vi "BMU参数读取-Auto.vi"(7 "Socket":dbl, 8 "CAN端口":u16(ring), 9 "设备索引号":u16(ring), 10 "CAN卡类型":u32(ring)=21, 11 "从板号":u8=1) -> (3 "成功?":bool)   [LabVIEW 2013] (continued)
                n2798 = global read "功能码全局.vi" "主板项目信息5"() -> (w4409:bool[])
                n2799 = global read "功能码全局.vi" "主板项目信息6"() -> (w4407:bool[])
                n2800 = Index Array(array=w4409, index=4 ("索引")) -> (element=w4405:bool)
                n2801 = Index Array(array=w4407, index=5 ("索引")) -> (element=w4406:bool)
                n2802 = Not(x=w4415) -> (.not. x?=w4414:bool)
              }
              frame "温度起始值" {
                w4451 = 2
                w4453 = FALSE
                n2803 = property on="电池实际容量(A)" class="DigNum (严格)"("Disabled"=w4451) -> ()  [unwired: 2 in, 2 out]
                n2804 = property on="使用者" class="DigNum (严格)"("Disabled"=w4451) -> ()  [unwired: 2 in, 2 out]
                n2805 = property on="SOH(%)" class="DigNum (严格)"("Disabled"=w4451) -> ()  [unwired: 2 in, 2 out]
                n2806 = property on="电池额定容量(A)" class="DigNum (严格)"("Disabled"=w4451) -> ()  [unwired: 2 in, 2 out]
                n2807 = property on="SOC(%)" class="DigNum (严格)"("Disabled"=w4451) -> ()  [unwired: 2 in, 2 out]
                n2808 = local read "从板个数"() -> (w4449:dbl)
                n2809 = property on="系统时钟" class="Str"("Disabled"=w4451) -> ()  [unwired: 2 in, 2 out]
                n2810 = property on="配置文件版本" class="Str"("Disabled"=w4451) -> ()  [unwired: 2 in, 2 out]
                n2811 = property on="车架(牌)号" class="Str"("Disabled"=w4451) -> ()  [unwired: 2 in, 2 out]
                n2812 = property on="产品编号" class="Str"("Disabled"=w4451) -> ()  [unwired: 2 in, 2 out]
                n2813 = control-ref of="项目信息"() -> (w4450:refnum<vi>)
                n2814 = stacked-sequence {
                  tunnel: w4450 -> [w4462 w4465 w4478]
                  tunnel: w4449 -> [w4455 w4464 w4477]
                  frame #0 {
                    n2815 = Multiply(x=w4455, y=3.0) -> (x*y=w4457:dbl)
                    n2816 = Compound Arithmetic op=ADD(23.0 ("值"), w4457) -> (w4459:dbl)
                    n2817 = Bundle(w4459, 0) -> (w4461:cluster{dbl, i32})  [unwired: 1 out]
                    n2818 = property class="Tbl (严格)"(reference=w4462, "Index Values"=w4461) -> ()  [unwired: 1 in, 2 out]
                  }
                  frame #1 {
                    n2819 = for {
                      N: 10 -> [_]
                      tunnel: w4465 -> [w4475]
                      tunnel: w4464 -> [w4470]
                      i -> [w4469]
                      n2820 = Multiply(x=4.0, y=w4470) -> (x*y=w4467:dbl)
                      n2821 = Compound Arithmetic op=ADD(24.0 ("值"), w4467, w4469) -> (w4472:dbl)
                      n2822 = Bundle(w4472, 0) -> (w4474:cluster{dbl, i32})  [unwired: 1 out]
                      n2823 = property class="Tbl (严格)"(reference=w4475, "Active Cell"=w4474, "Cell BG Color"=u32 16448250) -> ()  [unwired: 1 in, 2 out]
                    }
                  }
                  frame #2 {
                    n2824 = Increment(x=w4477) -> (x+1=w4476:dbl)
                    n2825 = for {
                      N: w4476 -> [_]
                      tunnel: w4478 -> [w4488]
                      tunnel: w4477 -> [w4483]
                      i -> [w4482]
                      n2826 = Multiply(x=3.0, y=w4483) -> (x*y=w4480:dbl)
                      n2827 = Compound Arithmetic op=ADD(23.0 ("值"), w4480, w4482) -> (w4485:dbl)
                      n2828 = Bundle(w4485, 0) -> (w4487:cluster{dbl, i32})  [unwired: 1 out]
                      n2829 = property class="Tbl (严格)"(reference=w4488, "Active Cell"=w4487, "Cell BG Color"=u32 6618880) -> ()  [unwired: 1 in, 2 out]
                    }
                  }
                }
                n2830 = Select(t=0, s=w4440, f=1) -> (s? t:f=w4439:i32)
                n2831 = property on="从板个数" class="DigNum (严格)"("NumText.BGColor"=u32 13816530) -> ()  [unwired: 2 in, 2 out]
                n2832 = property on="项目信息" class="Tbl (严格)"("Disabled"=w4439) -> ()  [unwired: 2 in, 2 out]
                n2833 = global read "功能码全局.vi" "主板项目信息5"() -> (w4447:bool[])
                n2834 = global read "功能码全局.vi" "主板项目信息6"() -> (w4445:bool[])
                n2835 = Index Array(array=w4447, index=5 ("索引")) -> (element=w4444:bool)
                n2836 = Index Array(array=w4445, index=6 ("索引")) -> (element=w4443:bool)
                n2837 = Not(x=w4453) -> (.not. x?=w4452:bool)
              }
              frame "保险位置" {
                w4501 = 2
                w4503 = FALSE
                n2838 = property on="电池实际容量(A)" class="DigNum (严格)"("Disabled"=w4501) -> ()  [unwired: 2 in, 2 out]
                n2839 = property on="使用者" class="DigNum (严格)"("Disabled"=w4501) -> ()  [unwired: 2 in, 2 out]
                n2840 = property on="SOH(%)" class="DigNum (严格)"("Disabled"=w4501) -> ()  [unwired: 2 in, 2 out]
                n2841 = property on="电池额定容量(A)" class="DigNum (严格)"("Disabled"=w4501) -> ()  [unwired: 2 in, 2 out]
                n2842 = property on="SOC(%)" class="DigNum (严格)"("Disabled"=w4501) -> ()  [unwired: 2 in, 2 out]
                n2843 = local read "从板个数"() -> (w4499:dbl)
                n2844 = property on="系统时钟" class="Str"("Disabled"=w4501) -> ()  [unwired: 2 in, 2 out]
                n2845 = property on="配置文件版本" class="Str"("Disabled"=w4501) -> ()  [unwired: 2 in, 2 out]
                n2846 = property on="车架(牌)号" class="Str"("Disabled"=w4501) -> ()  [unwired: 2 in, 2 out]
                n2847 = property on="产品编号" class="Str"("Disabled"=w4501) -> ()  [unwired: 2 in, 2 out]
                n2848 = control-ref of="项目信息"() -> (w4500:refnum<vi>)
                n2849 = stacked-sequence {
                  tunnel: w4500 -> [w4512 w4515]
                  tunnel: w4499 -> [w4505 w4514]
                  frame #0 {
                    n2850 = Multiply(x=w4505, y=4.0) -> (x*y=w4507:dbl)
                    n2851 = Compound Arithmetic op=ADD(24.0 ("值"), w4507) -> (w4509:dbl)
                    n2852 = Bundle(w4509, 0) -> (w4511:cluster{dbl, i32})  [unwired: 1 out]
                    n2853 = property class="Tbl (严格)"(reference=w4512, "Index Values"=w4511) -> ()  [unwired: 1 in, 2 out]
                  }
                  frame #1 {
                    n2854 = for {
                      N: 20 -> [_]
                      tunnel: w4515 -> [w4525]
                      tunnel: w4514 -> [w4520]
                      i -> [w4519]
                      n2855 = Multiply(x=4.0, y=w4520) -> (x*y=w4517:dbl)
                      n2856 = Compound Arithmetic op=ADD(24.0 ("值"), w4517, w4519) -> (w4522:dbl)
                      n2857 = Bundle(w4522, 0) -> (w4524:cluster{dbl, i32})  [unwired: 1 out]
                      n2858 = property class="Tbl (严格)"(reference=w4525, "Active Cell"=w4524, "Cell BG Color"=u32 6618880) -> ()  [unwired: 1 in, 2 out]
                    }
                  }
                }
                n2859 = property on="从板个数" class="DigNum (严格)"("NumText.BGColor"=u32 13816530) -> ()  [unwired: 2 in, 2 out]
                n2860 = Select(t=0, s=w4492, f=1) -> (s? t:f=w4490:i32)
                n2861 = global read "功能码全局.vi" "主板项目信息4"() -> (w4497:bool[])
                n2862 = property on="项目信息" class="Tbl (严格)"("Disabled"=w4490) -> ()  [unwired: 2 in, 2 out]
                n2863 = Index Array(array=w4497, index #1=5 ("索引"), index #2=6 ("索引")) -> (element #1=w4495:bool, element #2=w4494:bool)
                n2864 = Not(x=w4503) -> (.not. x?=w4502:bool)
              }
              frame "SOC" {
                w4536 = 2
                w4538 = FALSE
                n2865 = property on="电池实际容量(A)" class="DigNum (严格)"("Disabled"=w4536) -> ()  [unwired: 2 in, 2 out]
                n2866 = property on="使用者" class="DigNum (严格)"("Disabled"=w4536) -> ()  [unwired: 2 in, 2 out]
                n2867 = property on="SOH(%)" class="DigNum (严格)"("Disabled"=w4536) -> ()  [unwired: 2 in, 2 out]
                n2868 = property on="电池额定容量(A)" class="DigNum (严格)"("Disabled"=w4536) -> ()  [unwired: 2 in, 2 out]
                n2869 = property on="从板个数" class="DigNum (严格)"("NumText.BGColor"=u32 13816530) -> ()  [unwired: 2 in, 2 out]
                n2870 = property on="系统时钟" class="Str"("Disabled"=w4536) -> ()  [unwired: 2 in, 2 out]
                n2871 = property on="配置文件版本" class="Str"("Disabled"=w4536) -> ()  [unwired: 2 in, 2 out]
                n2872 = property on="车架(牌)号" class="Str"("Disabled"=w4536) -> ()  [unwired: 2 in, 2 out]
                n2873 = property on="项目信息" class="Tbl (严格)"("Disabled"=w4536) -> ()  [unwired: 2 in, 2 out]
                n2874 = property on="产品编号" class="Str"("Disabled"=w4536) -> ()  [unwired: 2 in, 2 out]
                n2875 = Select(t=0, s=w4528, f=0) -> (s? t:f=w4527:i32)
                n2876 = property on="SOC(%)" class="DigNum (严格)"("Disabled"=w4527) -> ()  [unwired: 2 in, 2 out]
                n2877 = property on="项目信息2" class="Clust (严格)"("DisabledEnum"=w4527) -> ()  [unwired: 2 in, 2 out]
                n2878 = global read "功能码全局.vi" "主板项目信息7"() -> (w4534:bool[])
                n2879 = Index Array(array=w4534, index #1=2 ("索引"), index #2=5 ("索引")) -> (element #1=w4532:bool, element #2=w4531:bool)
                n2880 = Not(x=w4538) -> (.not. x?=w4537:bool)
              }
              frame "电池额定实际容量" {
                w4550 = 2
                w4552 = FALSE
                n2881 = property on="使用者" class="DigNum (严格)"("Disabled"=w4550) -> ()  [unwired: 2 in, 2 out]
                n2882 = property on="SOH(%)" class="DigNum (严格)"("Disabled"=w4550) -> ()  [unwired: 2 in, 2 out]
                n2883 = property on="SOC(%)" class="DigNum (严格)"("Disabled"=w4550) -> ()  [unwired: 2 in, 2 out]
                n2884 = property on="从板个数" class="DigNum (严格)"("NumText.BGColor"=u32 13816530) -> ()  [unwired: 2 in, 2 out]
                n2885 = property on="系统时钟" class="Str"("Disabled"=w4550) -> ()  [unwired: 2 in, 2 out]
                n2886 = property on="配置文件版本" class="Str"("Disabled"=w4550) -> ()  [unwired: 2 in, 2 out]
                n2887 = property on="车架(牌)号" class="Str"("Disabled"=w4550) -> ()  [unwired: 2 in, 2 out]
                n2888 = property on="项目信息" class="Tbl (严格)"("Disabled"=w4550) -> ()  [unwired: 2 in, 2 out]
                n2889 = property on="产品编号" class="Str"("Disabled"=w4550) -> ()  [unwired: 2 in, 2 out]
                n2890 = Select(t=0, s=w4542, f=1) -> (s? t:f=w4541:i32)
                n2891 = property on="电池实际容量(A)" class="DigNum (严格)"("Disabled"=w4541) -> ()  [unwired: 2 in, 2 out]
                n2892 = property on="电池额定容量(A)" class="DigNum (严格)"("Disabled"=w4541) -> ()  [unwired: 2 in, 2 out]
                n2893 = property on="项目信息2" class="Clust (严格)"("DisabledEnum"=w4541) -> ()  [unwired: 2 in, 2 out]
                n2894 = global read "功能码全局.vi" "主板项目信息7"() -> (w4548:bool[])
                n2895 = Index Array(array=w4548, index #1=3 ("索引"), index #2=6 ("索引")) -> (element #1=w4546:bool, element #2=w4545:bool)
                n2896 = Not(x=w4552) -> (.not. x?=w4551:bool)
              }
              frame "配置文件版本" {
                w4565 = 2
                w4567 = FALSE
                n2897 = property on="使用者" class="DigNum (严格)"("Disabled"=w4565) -> ()  [unwired: 2 in, 2 out]
                n2898 = property on="SOH(%)" class="DigNum (严格)"("Disabled"=w4565) -> ()  [unwired: 2 in, 2 out]
                n2899 = property on="SOC(%)" class="DigNum (严格)"("Disabled"=w4565) -> ()  [unwired: 2 in, 2 out]
                n2900 = property on="电池实际容量(A)" class="DigNum (严格)"("Disabled"=w4565) -> ()  [unwired: 2 in, 2 out]
                n2901 = property on="从板个数" class="DigNum (严格)"("NumText.BGColor"=u32 13816530) -> ()  [unwired: 2 in, 2 out]
                n2902 = property on="电池额定容量(A)" class="DigNum (严格)"("Disabled"=w4565) -> ()  [unwired: 2 in, 2 out]
                n2903 = property on="系统时钟" class="Str"("Disabled"=w4565) -> ()  [unwired: 2 in, 2 out]
                n2904 = property on="车架(牌)号" class="Str"("Disabled"=w4565) -> ()  [unwired: 2 in, 2 out]
                n2905 = property on="项目信息" class="Tbl (严格)"("Disabled"=w4565) -> ()  [unwired: 2 in, 2 out]
                n2906 = property on="产品编号" class="Str"("Disabled"=w4565) -> ()  [unwired: 2 in, 2 out]
                n2907 = Select(t=0, s=w4556, f=1) -> (s? t:f=w4555:i32)
                n2908 = property on="项目信息2" class="Clust (严格)"("DisabledEnum"=w4555) -> ()  [unwired: 2 in, 2 out]
                n2909 = property on="配置文件版本" class="Str"("Disabled"=w4555) -> ()  [unwired: 2 in, 2 out]
                n2910 = global read "功能码全局.vi" "主板项目信息5"() -> (w4563:bool[])
                n2911 = global read "功能码全局.vi" "主板项目信息6"() -> (w4562:bool[])
                n2912 = Index Array(array=w4563, index=6 ("索引")) -> (element=w4560:bool)
                n2913 = Index Array(array=w4562, index=7 ("索引")) -> (element=w4559:bool)
                n2914 = Not(x=w4567) -> (.not. x?=w4566:bool)
              }
              frame "参数修改记录" {
                w4580 = 2
                w4582 = FALSE
                n2915 = property on="SOH(%)" class="DigNum (严格)"("Disabled"=w4580) -> ()  [unwired: 2 in, 2 out]
                n2916 = property on="SOC(%)" class="DigNum (严格)"("Disabled"=w4580) -> ()  [unwired: 2 in, 2 out]
                n2917 = property on="电池实际容量(A)" class="DigNum (严格)"("Disabled"=w4580) -> ()  [unwired: 2 in, 2 out]
                n2918 = property on="电池额定容量(A)" class="DigNum (严格)"("Disabled"=w4580) -> ()  [unwired: 2 in, 2 out]
                n2919 = property on="从板个数" class="DigNum (严格)"("NumText.BGColor"=u32 13816530) -> ()  [unwired: 2 in, 2 out]
                n2920 = property on="系统时钟" class="Str"("Disabled"=w4580) -> ()  [unwired: 2 in, 2 out]
                n2921 = property on="车架(牌)号" class="Str"("Disabled"=w4580) -> ()  [unwired: 2 in, 2 out]
                n2922 = property on="配置文件版本" class="Str"("Disabled"=w4580) -> ()  [unwired: 2 in, 2 out]
                n2923 = property on="项目信息" class="Tbl (严格)"("Disabled"=w4580) -> ()  [unwired: 2 in, 2 out]
                n2924 = property on="产品编号" class="Str"("Disabled"=w4580) -> ()  [unwired: 2 in, 2 out]
                n2925 = Select(t=0, s=w4571, f=1) -> (s? t:f=w4570:i32)
                n2926 = property on="使用者" class="DigNum (严格)"("Disabled"=w4570) -> ()  [unwired: 2 in, 2 out]
                n2927 = property on="项目信息2" class="Clust (严格)"("DisabledEnum"=w4570) -> ()  [unwired: 2 in, 2 out]
                n2928 = global read "功能码全局.vi" "主板项目信息7"() -> (w4577:bool[])
                n2929 = global read "功能码全局.vi" "主板项目信息5"() -> (w4578:bool[])
                n2930 = Index Array(array=w4577, index=0 ("索引")) -> (element=w4575:bool)
                n2931 = Index Array(array=w4578, index=7 ("索引")) -> (element=w4574:bool)
                n2932 = Not(x=w4582) -> (.not. x?=w4581:bool)
              }
              frame "车牌号" {
                w4595 = 2
                w4597 = FALSE
                n2933 = property on="SOH(%)" class="DigNum (严格)"("Disabled"=w4595) -> ()  [unwired: 2 in, 2 out]
                n2934 = property on="使用者" class="DigNum (严格)"("Disabled"=w4595) -> ()  [unwired: 2 in, 2 out]
                n2935 = property on="SOC(%)" class="DigNum (严格)"("Disabled"=w4595) -> ()  [unwired: 2 in, 2 out]
                n2936 = property on="电池实际容量(A)" class="DigNum (严格)"("Disabled"=w4595) -> ()  [unwired: 2 in, 2 out]
                n2937 = property on="电池额定容量(A)" class="DigNum (严格)"("Disabled"=w4595) -> ()  [unwired: 2 in, 2 out]
                n2938 = property on="从板个数" class="DigNum (严格)"("NumText.BGColor"=u32 13816530) -> ()  [unwired: 2 in, 2 out]
                n2939 = property on="系统时钟" class="Str"("Disabled"=w4595) -> ()  [unwired: 2 in, 2 out]
                n2940 = property on="配置文件版本" class="Str"("Disabled"=w4595) -> ()  [unwired: 2 in, 2 out]
                n2941 = property on="项目信息" class="Tbl (严格)"("Disabled"=w4595) -> ()  [unwired: 2 in, 2 out]
                n2942 = property on="产品编号" class="Str"("Disabled"=w4595) -> ()  [unwired: 2 in, 2 out]
                n2943 = Select(t=0, s=w4586, f=1) -> (s? t:f=w4585:i32)
                n2944 = property on="车架(牌)号" class="Str"("Disabled"=w4585) -> ()  [unwired: 2 in, 2 out]
                n2945 = property on="项目信息2" class="Clust (严格)"("DisabledEnum"=w4585) -> ()  [unwired: 2 in, 2 out]
                n2946 = global read "功能码全局.vi" "主板项目信息7"() -> (w4592:bool[])
                n2947 = global read "功能码全局.vi" "主板项目信息6"() -> (w4593:bool[])
                n2948 = Index Array(array=w4592, index=1 ("索引")) -> (element=w4590:bool)
                n2949 = Index Array(array=w4593, index=0 ("索引")) -> (element=w4589:bool)
                n2950 = Not(x=w4597) -> (.not. x?=w4596:bool)
              }
              frame "SOH" {
                w4609 = 2
                w4611 = FALSE
                n2951 = property on="使用者" class="DigNum (严格)"("Disabled"=w4609) -> ()  [unwired: 2 in, 2 out]
                n2952 = property on="SOC(%)" class="DigNum (严格)"("Disabled"=w4609) -> ()  [unwired: 2 in, 2 out]
                n2953 = property on="电池实际容量(A)" class="DigNum (严格)"("Disabled"=w4609) -> ()  [unwired: 2 in, 2 out]
                n2954 = property on="电池额定容量(A)" class="DigNum (严格)"("Disabled"=w4609) -> ()  [unwired: 2 in, 2 out]
                n2955 = property on="从板个数" class="DigNum (严格)"("NumText.BGColor"=u32 13816530) -> ()  [unwired: 2 in, 2 out]
                n2956 = property on="系统时钟" class="Str"("Disabled"=w4609) -> ()  [unwired: 2 in, 2 out]
                n2957 = property on="配置文件版本" class="Str"("Disabled"=w4609) -> ()  [unwired: 2 in, 2 out]
                n2958 = property on="项目信息" class="Tbl (严格)"("Disabled"=w4609) -> ()  [unwired: 2 in, 2 out]
                n2959 = property on="产品编号" class="Str"("Disabled"=w4609) -> ()  [unwired: 2 in, 2 out]
                n2960 = property on="车架(牌)号" class="Str"("Disabled"=w4609) -> ()  [unwired: 2 in, 2 out]
                n2961 = Select(t=0, s=w4601, f=1) -> (s? t:f=w4600:i32)
                n2962 = property on="项目信息2" class="Clust (严格)"("DisabledEnum"=w4600) -> ()  [unwired: 2 in, 2 out]
                n2963 = property on="SOH(%)" class="DigNum (严格)"("Disabled"=w4600) -> ()  [unwired: 2 in, 2 out]
                n2964 = global read "功能码全局.vi" "主板项目信息7"() -> (w4608:bool[])
                n2965 = Index Array(array=w4608, index #1=4 ("索引"), index #2=7 ("索引")) -> (element #1=w4605:bool, element #2=w4604:bool)
                n2966 = Not(x=w4611) -> (.not. x?=w4610:bool)
              }
              frame "SOC过低(2)", "SOC过高(2)", "SOH过低(2)", "充电电流过高(2)", "单体电压过低(2)", "单体电压过高(2)", "单组电压不均衡(2)", "单组温度不均衡(2)", "二级故障阀值", "放电电流过高(2)", "极柱温度过高(2)", "内阻过大(2)", "温度过低(2)", "温度过高(2)", "整组电压不均衡(2)", "整组温度不均衡(2)", "总电压过低(2)", "总电压过高(2)" {
                w4623 = FALSE
                n2967 = property on="从板个数" class="DigNum (严格)"("NumText.BGColor"=u32 13816530) -> ()  [unwired: 2 in, 2 out]
                n2968 = Select(t=0, s=w4615, f=1) -> (s? t:f=w4614:i32)
                n2969 = property on="一级故障 2" class="Clust (严格)"("DisabledEnum"=w4614) -> ()  [unwired: 2 in, 2 out]
                n2970 = global read "功能码全局.vi" "主板故障阀值9"() -> (w4621:bool[])
                n2971 = Index Array(array=w4621, index #1=3 ("索引"), index #2=6 ("索引")) -> (element #1=w4619:bool, element #2=w4618:bool)
                n2972 = Not(x=w4623) -> (.not. x?=w4624:bool)
              }
              frame "SOC过低(3)", "SOC过高(3)", "SOH过低(3)", "充电电流过高(3)", "单体电压过低(3)", "单体电压过高(3)", "单组电压不均衡(3)", "单组温度不均衡(3)", "放电电流过高(3)", "极柱温度过高(3)", "内阻过大(3)", "三级故障阀值", "温度过低(3)", "温度过高(3)", "整组电压不均衡(3)", "整组温度不均衡(3)", "总电压过低(3)", "总电压过高(3)" {
                w4637 = FALSE
                n2973 = property on="从板个数" class="DigNum (严格)"("NumText.BGColor"=u32 13816530) -> ()  [unwired: 2 in, 2 out]
                n2974 = Select(t=0, s=w4628, f=1) -> (s? t:f=w4627:i32)
                n2975 = property on="一级故障 3" class="Clust (严格)"("DisabledEnum"=w4627) -> ()  [unwired: 2 in, 2 out]
                n2976 = global read "功能码全局.vi" "主板故障阀值9"() -> (w4634:bool[])
                n2977 = Index Array(array=w4634, index #1=4 ("索引"), index #2=7 ("索引")) -> (element #1=w4632:bool, element #2=w4631:bool)
                n2978 = Not(x=w4637) -> (.not. x?=w4636:bool)
              }
              frame "SOC过低", "SOC过高", "SOH过低", "充电电流过高", "单体电压过低", "单体电压过高", "单组电压不均衡", "单组温度不均衡", "放电电流过高", "极柱温度过高", "内阻过大", "温度过低", "温度过高", "一级故障阀值", "整组电压不均衡", "整组温度不均衡", "总电压过低", "总电压过高" {
                w4650 = FALSE
                n2979 = Select(t=0, s=w4641, f=1) -> (s? t:f=w4640:i32)
                n2980 = property on="从板个数" class="DigNum (严格)"("NumText.BGColor"=u32 13816530) -> ()  [unwired: 2 in, 2 out]
                n2981 = property on="一级故障" class="Clust (严格)"("DisabledEnum"=w4640) -> ()  [unwired: 2 in, 2 out]
                n2982 = global read "功能码全局.vi" "主板故障阀值9"() -> (w4647:bool[])
                n2983 = Index Array(array=w4647, index #1=2 ("索引"), index #2=5 ("索引")) -> (element #1=w4645:bool, element #2=w4644:bool)
                n2984 = Not(x=w4650) -> (.not. x?=w4649:bool)
              }
              frame "充电控制参数", "电流步长", "最大允许充电电流", "最大允许充电温度", "最大允许单体电压", "最大允许总电压", "最小允许充电电流", "最小允许充电温度", "最小允许单体电压" {
                w4653 = 2
                w4664 = FALSE
                n2985 = property on="从板个数" class="DigNum (严格)"("NumText.BGColor"=u32 13816530) -> ()  [unwired: 2 in, 2 out]
                n2986 = property on="风机开启温度" class="DigNum (严格)"("Disabled"=w4653) -> ()  [unwired: 2 in, 2 out]
                n2987 = property on="风机关闭温度" class="DigNum (严格)"("Disabled"=w4653) -> ()  [unwired: 2 in, 2 out]
                n2988 = property on="加热开启温度" class="DigNum (严格)"("Disabled"=w4653) -> ()  [unwired: 2 in, 2 out]
                n2989 = property on="加热关闭温度" class="DigNum (严格)"("Disabled"=w4653) -> ()  [unwired: 2 in, 2 out]
                n2990 = property on="风机开启温差" class="DigNum (严格)"("Disabled"=w4653) -> ()  [unwired: 2 in, 2 out]
                n2991 = property on="风机关闭温差" class="DigNum (严格)"("Disabled"=w4653) -> ()  [unwired: 2 in, 2 out]
                n2992 = property on="加热控制参数" class="Clust (严格)"("DisabledEnum"=w4653) -> ()  [unwired: 2 in, 2 out]
                n2993 = Select(t=0, s=w4655, f=1) -> (s? t:f=w4654:i32)
                n2994 = property on="最大允许总电压" class="DigNum (严格)"("Disabled"=w4654) -> ()  [unwired: 2 in, 2 out]
                n2995 = property on="最大允许充电温度" class="DigNum (严格)"("Disabled"=w4654) -> ()  [unwired: 2 in, 2 out]
                n2996 = property on="最小允许充电温度" class="DigNum (严格)"("Disabled"=w4654) -> ()  [unwired: 2 in, 2 out]
                n2997 = property on="电流步长" class="DigNum (严格)"("Disabled"=w4654) -> ()  [unwired: 2 in, 2 out]
                n2998 = property on="最大允许单体电压" class="DigNum (严格)"("Disabled"=w4654) -> ()  [unwired: 2 in, 2 out]
                n2999 = property on="最小允许单体电压" class="DigNum (严格)"("Disabled"=w4654) -> ()  [unwired: 2 in, 2 out]
                n3000 = property on="最大允许充电电流" class="DigNum (严格)"("Disabled"=w4654) -> ()  [unwired: 2 in, 2 out]
                n3001 = property on="最小允许充电电流" class="DigNum (严格)"("Disabled"=w4654) -> ()  [unwired: 2 in, 2 out]
                n3002 = global read "功能码全局.vi" "主板控制类信息10"() -> (w4661:bool[])
                n3003 = Index Array(array=w4661, index #1=5 ("索引"), index #2=7 ("索引")) -> (element #1=w4659:bool, element #2=w4658:bool)
                n3004 = Not(x=w4664) -> (.not. x?=w4663:bool)
              }
              frame "风机关闭温差", "风机关闭温度", "风机开启温差", "风机开启温度", "加热关闭温差", "加热关闭温度", "加热开启温度", "加热控制参数" {
                w4676 = 2
                w4678 = FALSE
                n3005 = Select(t=0, s=w4668, f=1) -> (s? t:f=w4667:i32)
                n3006 = property on="从板个数" class="DigNum (严格)"("NumText.BGColor"=u32 13816530) -> ()  [unwired: 2 in, 2 out]
                n3007 = property on="加热控制参数" class="Clust (严格)"("DisabledEnum"=w4667) -> ()  [unwired: 2 in, 2 out]
                n3008 = property on="风机开启温度" class="DigNum (严格)"("Disabled"=w4667) -> ()  [unwired: 2 in, 2 out]
                n3009 = property on="风机关闭温度" class="DigNum (严格)"("Disabled"=w4667) -> ()  [unwired: 2 in, 2 out]
                n3010 = property on="加热开启温度" class="DigNum (严格)"("Disabled"=w4667) -> ()  [unwired: 2 in, 2 out]
                n3011 = property on="加热关闭温度" class="DigNum (严格)"("Disabled"=w4667) -> ()  [unwired: 2 in, 2 out]
                n3012 = property on="风机开启温差" class="DigNum (严格)"("Disabled"=w4667) -> ()  [unwired: 2 in, 2 out]
                n3013 = property on="风机关闭温差" class="DigNum (严格)"("Disabled"=w4667) -> ()  [unwired: 2 in, 2 out]
                n3014 = property on="最大允许总电压" class="DigNum (严格)"("Disabled"=w4676) -> ()  [unwired: 2 in, 2 out]
                n3015 = property on="最大允许充电温度" class="DigNum (严格)"("Disabled"=w4676) -> ()  [unwired: 2 in, 2 out]
                n3016 = property on="最小允许充电温度" class="DigNum (严格)"("Disabled"=w4676) -> ()  [unwired: 2 in, 2 out]
                n3017 = property on="电流步长" class="DigNum (严格)"("Disabled"=w4676) -> ()  [unwired: 2 in, 2 out]
                n3018 = property on="最大允许单体电压" class="DigNum (严格)"("Disabled"=w4676) -> ()  [unwired: 2 in, 2 out]
                n3019 = property on="最小允许单体电压" class="DigNum (严格)"("Disabled"=w4676) -> ()  [unwired: 2 in, 2 out]
                n3020 = property on="最大允许充电电流" class="DigNum (严格)"("Disabled"=w4676) -> ()  [unwired: 2 in, 2 out]
                n3021 = property on="最小允许充电电流" class="DigNum (严格)"("Disabled"=w4676) -> ()  [unwired: 2 in, 2 out]
                n3022 = global read "功能码全局.vi" "主板控制类信息10"() -> (w4674:bool[])
                n3023 = Index Array(array=w4674, index #1=4 ("索引"), index #2=6 ("索引")) -> (element #1=w4672:bool, element #2=w4671:bool)
                n3024 = Not(x=w4678) -> (.not. x?=w4677:bool)
              }
              frame "电池信息" {
                w4691 = FALSE
                n3025 = Select(t=0, s=w4682, f=1) -> (s? t:f=w4681:i32)
                n3026 = property on="电池串联" class="DigNum (严格)"("Disabled"=w4681) -> ()  [unwired: 2 in, 2 out]
                n3027 = property on="电池并联" class="DigNum (严格)"("Disabled"=w4681) -> ()  [unwired: 2 in, 2 out]
                n3028 = property on="电池包额定容量" class="DigNum (严格)"("Disabled"=w4681) -> ()  [unwired: 2 in, 2 out]
                n3029 = property on="电池包额定能量(kWh)" class="DigNum (严格)"("Disabled"=w4681) -> ()  [unwired: 2 in, 2 out]
                n3030 = property on="电池包额定总电压" class="DigNum (严格)"("Disabled"=w4681) -> ()  [unwired: 2 in, 2 out]
                n3031 = property on="实际容量" class="DigNum (严格)"("Disabled"=w4681) -> ()  [unwired: 2 in, 2 out]
                n3032 = property on="电池包组号" class="Str"("Disabled"=w4681) -> ()  [unwired: 2 in, 2 out]
                n3033 = property on="电池生产日期" class="Str"("Disabled"=w4681) -> ()  [unwired: 2 in, 2 out]
                n3034 = property on="电池厂家" class="Str"("Disabled"=w4681) -> ()  [unwired: 2 in, 2 out]
                n3035 = property on="电池类型" class="Str"("Disabled"=w4681) -> ()  [unwired: 2 in, 2 out]
                n3036 = property on="累计充电总安时" class="DigNum (严格)"("Disabled"=w4681) -> ()  [unwired: 2 in, 2 out]
                n3037 = property on="累计放电总安时" class="DigNum (严格)"("Disabled"=w4681) -> ()  [unwired: 2 in, 2 out]
                n3038 = property on="电池放空次数" class="DigNum (严格)"("Disabled"=w4681) -> ()  [unwired: 2 in, 2 out]
                n3039 = property on="电池充满次数" class="DigNum (严格)"("Disabled"=w4681) -> ()  [unwired: 2 in, 2 out]
                n3040 = property on="电池充电次数" class="DigNum (严格)"("Disabled"=w4681) -> ()  [unwired: 2 in, 2 out]
                n3041 = property on="电池信息" class="Clust (严格)"("DisabledEnum"=w4681) -> ()  [unwired: 2 in, 2 out]
                n3042 = global read "功能码全局.vi" "主板版本号11"() -> (w4688:bool[])
                n3043 = property on="从板个数" class="DigNum (严格)"("NumText.BGColor"=u32 13816530) -> ()  [unwired: 2 in, 2 out]
                n3044 = Index Array(array=w4688, index #1=0 ("索引"), index #2=1 ("索引")) -> (element #1=w4686:bool, element #2=w4685:bool)
                n3045 = Not(x=w4691) -> (.not. x?=w4690:bool)
              }
              frame "电池信息1" {
                w4703 = 2
                w4705 = FALSE
                n3046 = Select(t=0, s=w4695, f=1) -> (s? t:f=w4694:i32)
                n3047 = property on="电池信息" class="Clust (严格)"("DisabledEnum"=w4694) -> ()  [unwired: 2 in, 2 out]
                n3048 = property on="电池生产日期" class="Str"("Disabled"=w4694) -> ()  [unwired: 2 in, 2 out]
                n3049 = property on="电池厂家" class="Str"("Disabled"=w4694) -> ()  [unwired: 2 in, 2 out]
                n3050 = property on="电池类型" class="Str"("Disabled"=w4694) -> ()  [unwired: 2 in, 2 out]
                n3051 = property on="电池串联" class="DigNum (严格)"("Disabled"=w4694) -> ()  [unwired: 2 in, 2 out]
                n3052 = property on="电池并联" class="DigNum (严格)"("Disabled"=w4694) -> ()  [unwired: 2 in, 2 out]
                n3053 = property on="电池包额定容量" class="DigNum (严格)"("Disabled"=w4694) -> ()  [unwired: 2 in, 2 out]
                n3054 = property on="电池包额定能量(kWh)" class="DigNum (严格)"("Disabled"=w4694) -> ()  [unwired: 2 in, 2 out]
                n3055 = property on="电池包额定总电压" class="DigNum (严格)"("Disabled"=w4694) -> ()  [unwired: 2 in, 2 out]
                n3056 = property on="实际容量" class="DigNum (严格)"("Disabled"=w4694) -> ()  [unwired: 2 in, 2 out]
                n3057 = property on="累计充电总安时" class="DigNum (严格)"("Disabled"=w4703) -> ()  [unwired: 2 in, 2 out]
                n3058 = property on="累计放电总安时" class="DigNum (严格)"("Disabled"=w4703) -> ()  [unwired: 2 in, 2 out]
                n3059 = property on="电池放空次数" class="DigNum (严格)"("Disabled"=w4703) -> ()  [unwired: 2 in, 2 out]
                n3060 = property on="电池充满次数" class="DigNum (严格)"("Disabled"=w4703) -> ()  [unwired: 2 in, 2 out]
                n3061 = property on="电池充电次数" class="DigNum (严格)"("Disabled"=w4703) -> ()  [unwired: 2 in, 2 out]
                n3062 = property on="从板个数" class="DigNum (严格)"("NumText.BGColor"=u32 13816530) -> ()  [unwired: 2 in, 2 out]
                n3063 = property on="电池包组号" class="Str"("Disabled"=w4703) -> ()  [unwired: 2 in, 2 out]
                n3064 = global read "功能码全局.vi" "主板版本号11"() -> (w4701:bool[])
                n3065 = Index Array(array=w4701, index #1=0 ("索引"), index #2=1 ("索引")) -> (element #1=w4699:bool, element #2=w4698:bool)
                n3066 = Not(x=w4705) -> (.not. x?=w4704:bool)
              }
              frame "电池包组号" {
                w4717 = 2
                w4719 = FALSE
                n3067 = property on="电池生产日期" class="Str"("Disabled"=w4717) -> ()  [unwired: 2 in, 2 out]
                n3068 = property on="电池厂家" class="Str"("Disabled"=w4717) -> ()  [unwired: 2 in, 2 out]
                n3069 = property on="电池类型" class="Str"("Disabled"=w4717) -> ()  [unwired: 2 in, 2 out]
                n3070 = property on="电池串联" class="DigNum (严格)"("Disabled"=w4717) -> ()  [unwired: 2 in, 2 out]
                n3071 = property on="电池并联" class="DigNum (严格)"("Disabled"=w4717) -> ()  [unwired: 2 in, 2 out]
                n3072 = property on="电池包额定容量" class="DigNum (严格)"("Disabled"=w4717) -> ()  [unwired: 2 in, 2 out]
                n3073 = property on="电池包额定能量(kWh)" class="DigNum (严格)"("Disabled"=w4717) -> ()  [unwired: 2 in, 2 out]
                n3074 = property on="电池包额定总电压" class="DigNum (严格)"("Disabled"=w4717) -> ()  [unwired: 2 in, 2 out]
                n3075 = property on="实际容量" class="DigNum (严格)"("Disabled"=w4717) -> ()  [unwired: 2 in, 2 out]
                n3076 = property on="从板个数" class="DigNum (严格)"("NumText.BGColor"=u32 13816530) -> ()  [unwired: 2 in, 2 out]
                n3077 = property on="累计充电总安时" class="DigNum (严格)"("Disabled"=w4717) -> ()  [unwired: 2 in, 2 out]
                n3078 = property on="累计放电总安时" class="DigNum (严格)"("Disabled"=w4717) -> ()  [unwired: 2 in, 2 out]
                n3079 = property on="电池放空次数" class="DigNum (严格)"("Disabled"=w4717) -> ()  [unwired: 2 in, 2 out]
                n3080 = property on="电池充满次数" class="DigNum (严格)"("Disabled"=w4717) -> ()  [unwired: 2 in, 2 out]
                n3081 = property on="电池充电次数" class="DigNum (严格)"("Disabled"=w4717) -> ()  [unwired: 2 in, 2 out]
                n3082 = Select(t=0, s=w4709, f=1) -> (s? t:f=w4708:i32)
                n3083 = property on="电池包组号" class="Str"("Disabled"=w4708) -> ()  [unwired: 2 in, 2 out]
                n3084 = property on="电池信息" class="Clust (严格)"("DisabledEnum"=w4708) -> ()  [unwired: 2 in, 2 out]
                n3085 = global read "功能码全局.vi" "主板版本号11"() -> (w4715:bool[])
                n3086 = Index Array(array=w4715, index #1=0 ("索引"), index #2=1 ("索引")) -> (element #1=w4713:bool, element #2=w4712:bool)
                n3087 = Not(x=w4719) -> (.not. x?=w4718:bool)
              }
              frame "充放电安时" {
                w4731 = 2
                w4733 = FALSE
                n3088 = property on="电池生产日期" class="Str"("Disabled"=w4731) -> ()  [unwired: 2 in, 2 out]
                n3089 = property on="电池厂家" class="Str"("Disabled"=w4731) -> ()  [unwired: 2 in, 2 out]
                n3090 = property on="电池类型" class="Str"("Disabled"=w4731) -> ()  [unwired: 2 in, 2 out]
                n3091 = property on="电池串联" class="DigNum (严格)"("Disabled"=w4731) -> ()  [unwired: 2 in, 2 out]
                n3092 = property on="电池并联" class="DigNum (严格)"("Disabled"=w4731) -> ()  [unwired: 2 in, 2 out]
                n3093 = property on="电池包额定容量" class="DigNum (严格)"("Disabled"=w4731) -> ()  [unwired: 2 in, 2 out]
                n3094 = property on="电池包额定能量(kWh)" class="DigNum (严格)"("Disabled"=w4731) -> ()  [unwired: 2 in, 2 out]
                n3095 = property on="电池包额定总电压" class="DigNum (严格)"("Disabled"=w4731) -> ()  [unwired: 2 in, 2 out]
                n3096 = property on="实际容量" class="DigNum (严格)"("Disabled"=w4731) -> ()  [unwired: 2 in, 2 out]
                n3097 = property on="从板个数" class="DigNum (严格)"("NumText.BGColor"=u32 13816530) -> ()  [unwired: 2 in, 2 out]
                n3098 = Select(t=0, s=w4723, f=1) -> (s? t:f=w4722:i32)
                n3099 = property on="电池放空次数" class="DigNum (严格)"("Disabled"=w4731) -> ()  [unwired: 2 in, 2 out]
                n3100 = property on="电池充满次数" class="DigNum (严格)"("Disabled"=w4731) -> ()  [unwired: 2 in, 2 out]
                n3101 = property on="电池充电次数" class="DigNum (严格)"("Disabled"=w4731) -> ()  [unwired: 2 in, 2 out]
                n3102 = property on="电池包组号" class="Str"("Disabled"=w4731) -> ()  [unwired: 2 in, 2 out]
                n3103 = property on="累计充电总安时" class="DigNum (严格)"("Disabled"=w4722) -> ()  [unwired: 2 in, 2 out]
                n3104 = property on="累计放电总安时" class="DigNum (严格)"("Disabled"=w4722) -> ()  [unwired: 2 in, 2 out]
                n3105 = property on="电池信息" class="Clust (严格)"("DisabledEnum"=w4722) -> ()  [unwired: 2 in, 2 out]
                n3106 = global read "功能码全局.vi" "主板版本号11"() -> (w4729:bool[])
                n3107 = Index Array(array=w4729, index #1=0 ("索引"), index #2=1 ("索引")) -> (element #1=w4727:bool, element #2=w4726:bool)
                n3108 = Not(x=w4733) -> (.not. x?=w4732:bool)
              }
              frame "电池充放电次数" {
                w4745 = 2
                w4747 = FALSE
                n3109 = property on="从板个数" class="DigNum (严格)"("NumText.BGColor"=u32 13816530) -> ()  [unwired: 2 in, 2 out]
                n3110 = property on="电池生产日期" class="Str"("Disabled"=w4745) -> ()  [unwired: 2 in, 2 out]
                n3111 = property on="电池厂家" class="Str"("Disabled"=w4745) -> ()  [unwired: 2 in, 2 out]
                n3112 = property on="电池类型" class="Str"("Disabled"=w4745) -> ()  [unwired: 2 in, 2 out]
                n3113 = property on="电池串联" class="DigNum (严格)"("Disabled"=w4745) -> ()  [unwired: 2 in, 2 out]
                n3114 = property on="电池并联" class="DigNum (严格)"("Disabled"=w4745) -> ()  [unwired: 2 in, 2 out]
                n3115 = property on="电池包额定容量" class="DigNum (严格)"("Disabled"=w4745) -> ()  [unwired: 2 in, 2 out]
                n3116 = property on="电池包额定能量(kWh)" class="DigNum (严格)"("Disabled"=w4745) -> ()  [unwired: 2 in, 2 out]
                n3117 = property on="电池包额定总电压" class="DigNum (严格)"("Disabled"=w4745) -> ()  [unwired: 2 in, 2 out]
                n3118 = property on="实际容量" class="DigNum (严格)"("Disabled"=w4745) -> ()  [unwired: 2 in, 2 out]
                n3119 = Select(t=0, s=w4737, f=1) -> (s? t:f=w4736:i32)
                n3120 = property on="电池放空次数" class="DigNum (严格)"("Disabled"=w4736) -> ()  [unwired: 2 in, 2 out]
                n3121 = property on="电池充满次数" class="DigNum (严格)"("Disabled"=w4736) -> ()  [unwired: 2 in, 2 out]
                n3122 = property on="电池充电次数" class="DigNum (严格)"("Disabled"=w4736) -> ()  [unwired: 2 in, 2 out]
                n3123 = property on="累计充电总安时" class="DigNum (严格)"("Disabled"=w4745) -> ()  [unwired: 2 in, 2 out]
                n3124 = property on="累计放电总安时" class="DigNum (严格)"("Disabled"=w4745) -> ()  [unwired: 2 in, 2 out]
                n3125 = property on="电池信息" class="Clust (严格)"("DisabledEnum"=w4736) -> ()  [unwired: 2 in, 2 out]
                n3126 = property on="电池包组号" class="Str"("Disabled"=w4745) -> ()  [unwired: 2 in, 2 out]
                n3127 = global read "功能码全局.vi" "主板版本号11"() -> (w4743:bool[])
                n3128 = Index Array(array=w4743, index #1=0 ("索引"), index #2=1 ("索引")) -> (element #1=w4741:bool, element #2=w4740:bool)
                n3129 = Not(x=w4747) -> (.not. x?=w4746:bool)
              }
              frame "假", Default {
                w4752 = FALSE
                n3130 = Not(x=w4752) -> (.not. x?=w4751:bool)
              }
            }
            n3131 = property on="单个读取" class="Bool (严格)"("Visible"=w4220) -> ()  [unwired: 2 in, 2 out]
            n3132 = property on="单个写入" class="Bool (严格)"("Visible"=w4219) -> ()  [unwired: 2 in, 2 out]
            n3133 = local write "1"(w4227) -> ()
            n3134 = local write "1 2"(w4226) -> ()
            n3135 = local write "1 3"(w4225) -> ()
            n3136 = local write "1 4"(w4224) -> ()
            n3137 = local write "1 5"(w4223) -> ()
            n3138 = local write "1 11"(w4222) -> ()
            n3139 = local write "主板2"(w4228) -> ()
          }
          event "从板选项": Mouse Down {
            n3140 = event-data() -> ("CtlRef"=w4767:refnum<vi>)  [unwired: 8 out]
            n3141 = property class="Tree (严格)"(reference=w4767) -> ("Value"=w4766:string)  [unwired: 1 in, 2 out]
            n3142 = global read "功能码全局.vi" "主板监控2"() -> (w4757:bool[])
            n3143 = Index Array(array=w4757, index=6 ("索引")) -> (element=w4755:bool)
            n3144 = case shown="\"二维码\"" w4766 {
              tunnel: [T20."从板信息" ("等级 2") T20."从板信息" ("等级 2") T20."从板信息" ("等级 2") T20."从板信息" ("等级 2") T20."从板信息" ("等级 2") T20."从板信息" ("等级 2") T20."从板信息" ("等级 2") T20."从板信息" ("等级 2") T20."一级故障阀值" ("等级 2") T20."二级故障阀值" ("等级 2") T20."三级故障阀值" ("等级 2") T20."快换参数" ("等级 2") T20."快换参数" ("等级 2") T20."快换参数" ("等级 2") T20."快换参数" ("等级 2") T20."快换参数" ("等级 2") T20."快换参数" ("等级 2") T20."快换参数" ("等级 2") T20."快换参数" ("等级 2") T15."均衡参数" ("等级 2") T15."均衡参数" ("等级 2") T15."均衡参数" ("等级 2") T20."从板信息" ("等级 2")] -> w4765
              tunnel: [w4778 w4788 w4798 w4812 w4827 w4862 w4899 w4936 w4960 w4973 w4986 w4999 w5025 w5039 w5055 w5072 w5089 w5107 w5126 w5143 w5156 w5170 w5185] -> w4764
              tunnel: [w4770 w4780 w4790 w4800 w4814 w4849 w4886 w4923 w4971 w4973 w4986 w4999 w5025 w5039 w5055 w5072 w5089 w5107 w5126 w5143 w5156 w5170 w5184] -> w4763
              tunnel: [w4770 w4780 w4790 w4800 w4814 w4849 w4886 w4923 w4960 w4984 w4986 w4999 w5025 w5039 w5055 w5072 w5089 w5107 w5126 w5143 w5156 w5170 w5184] -> w4762
              tunnel: [w4770 w4780 w4790 w4800 w4814 w4849 w4886 w4923 w4960 w4973 w4997 w4999 w5025 w5039 w5055 w5072 w5089 w5107 w5126 w5143 w5156 w5170 w5184] -> w4761
              tunnel: [w4770 w4780 w4790 w4800 w4814 w4849 w4886 w4923 w4960 w4973 w4986 w5023 w5037 w5053 w5070 w5087 w5105 w5124 w5141 w5143 w5156 w5170 w5184] -> w4760
              tunnel: [w4775 w4785 w4791 w4807 w4821 w4856 w4893 w4930 w4967 w4980 w4993 w5008 w5030 w5045 w5059 w5077 w5092 w5112 w5130 w5146 w5160 w5175 w5184] -> w4759
              tunnel: [w4772 w4782 w4791 w4806 w4820 w4855 w4892 w4929 w4966 w4979 w4992 w5000 w5029 w5044 w5058 w5078 w5093 w5111 w5129 w5145 w5159 w5174 w5184] -> w4758
              tunnel: w4755 -> [_ _ w4795 w4803 w4817 w4852 w4889 w4926 w4962 w4976 w4989 w5020 w5033 w5048 w5063 w5081 w5097 w5115 w5134 w5149 w5163 w5177 _]
              tunnel: [w4770 w4780 w4790 w4800 w4814 w4849 w4886 w4923 w4960 w4973 w4986 w4999 w5025 w5039 w5055 w5072 w5089 w5107 w5126 w5144 w5157 w5171 w5184] -> w4754
              frame "从板号" {
                w4777 = 2
                w4770 = FALSE ("1 6")
                n3145 = property on="项目信息 2" class="Tbl (严格)"("Disabled"=w4777) -> ()  [unwired: 2 in, 2 out]
                n3146 = property on="加热控制参数" class="Clust (严格)"("Disabled"=w4777) -> ()  [unwired: 2 in, 2 out]
                n3147 = property on="从板号" class="DigNum (严格)"("NumText.BGColor"=u32 6618880) -> ()  [unwired: 2 in, 2 out]
                n3148 = global read "功能码全局.vi" "16"() -> (w4774:bool[])
                n3149 = Index Array(array=w4774, index #1=4 ("索引"), index #2=6 ("索引")) -> (element #1=w4775:bool, element #2=w4772:bool)
                n3150 = Not(x=w4770) -> (.not. x?=w4778:bool)
              }
              frame "二维码" {
                w4787 = 2
                w4780 = FALSE ("1 6")
                n3151 = property on="项目信息 2" class="Tbl (严格)"("Disabled"=w4787) -> ()  [unwired: 2 in, 2 out]
                n3152 = property on="加热控制参数" class="Clust (严格)"("Disabled"=w4787) -> ()  [unwired: 2 in, 2 out]
                n3153 = property on="从板号" class="DigNum (严格)"("NumText.BGColor"=u32 6618880) -> ()  [unwired: 2 in, 2 out]
                n3154 = global read "功能码全局.vi" "16"() -> (w4784:bool[])
                n3155 = Index Array(array=w4784, index #1=4 ("索引"), index #2=6 ("索引")) -> (element #1=w4785:bool, element #2=w4782:bool)
                n3156 = Not(x=w4780) -> (.not. x?=w4788:bool)
              }
              frame "从板信息" {
                w4790 = FALSE ("1 6")
                n3157 = Select(t=0, s=w4795, f=1) -> (s? t:f=w4794:i32)
                n3158 = property on="从板号" class="DigNum (严格)"("NumText.BGColor"=u32 16777215) -> ()  [unwired: 2 in, 2 out]
                n3159 = property on="项目信息 2" class="Tbl (严格)"("Disabled"=w4794) -> ()  [unwired: 2 in, 2 out]
                n3160 = property on="加热控制参数" class="Clust (严格)"("Disabled"=w4794) -> ()  [unwired: 2 in, 2 out]
                n3161 = Not(x=w4790) -> (.not. x?=w4798:bool)
                n3162 = local read "从板项目信息"() -> (w4792:bool)
                n3163 = Not(x=w4792) -> (.not. x?=w4791:bool)
              }
              frame "风机关闭温差", "风机关闭温度", "风机开启温差", "风机开启温度", "加热关闭温差", "加热关闭温度", "加热开启温度", "加热控制参数" {
                w4800 = FALSE ("1 6")
                n3164 = property on="从板号" class="DigNum (严格)"("NumText.BGColor"=u32 16777215) -> ()  [unwired: 2 in, 2 out]
                n3165 = Select(t=0, s=w4803, f=1) -> (s? t:f=w4802:i32)
                n3166 = property on="项目信息 2" class="Tbl (严格)"("Disabled"=2) -> ()  [unwired: 2 in, 2 out]
                n3167 = property on="加热控制参数" class="Clust (严格)"("Disabled"=w4802) -> ()  [unwired: 2 in, 2 out]
                n3168 = global read "功能码全局.vi" "16"() -> (w4809:bool[])
                n3169 = Index Array(array=w4809, index #1=5 ("索引"), index #2=7 ("索引")) -> (element #1=w4807:bool, element #2=w4806:bool)
                n3170 = Not(x=w4800) -> (.not. x?=w4812:bool)
              }
              frame "电压个数" {
                w4814 = FALSE ("1 6")
                n3171 = property on="从板号" class="DigNum (严格)"("NumText.BGColor"=u32 16777215) -> ()  [unwired: 2 in, 2 out]
                n3172 = control-ref of="项目信息 2"() -> (w4825:refnum<vi>)
                n3173 = stacked-sequence {
                  tunnel: w4825 -> [w4832 w4834 w4843]
                  frame #0 {
                    n3174 = Bundle(0, 0) -> (w4831:cluster{i32, i32})  [unwired: 1 out]
                    n3175 = property class="Tbl (严格)"(reference=w4832, "Index Values"=w4831) -> ()  [unwired: 1 in, 2 out]
                  }
                  frame #1 {
                    n3176 = for {
                      N: 40 -> [_]
                      tunnel: w4834 -> [w4841]
                      i -> [w4836]
                      n3177 = Compound Arithmetic op=ADD(0 ("值"), w4836) -> (w4838:i32)
                      n3178 = Bundle(w4838, 0) -> (w4840:cluster{i32, i32})  [unwired: 1 out]
                      n3179 = property class="Tbl (严格)"(reference=w4841, "Active Cell"=w4840, "Cell BG Color"=u32 16448250) -> ()  [unwired: 1 in, 2 out]
                    }
                  }
                  frame #2 {
                    n3180 = for {
                      N: 1 -> [_]
                      tunnel: w4843 -> [w4848]
                      i -> [w4844]
                      n3181 = Bundle(w4844, 0) -> (w4847:cluster{i32, i32})  [unwired: 1 out]
                      n3182 = property class="Tbl (严格)"(reference=w4848, "Active Cell"=w4847, "Cell BG Color"=u32 6618880) -> ()  [unwired: 1 in, 2 out]
                    }
                  }
                }
                n3183 = Select(t=0, s=w4817, f=1) -> (s? t:f=w4816:i32)
                n3184 = property on="项目信息 2" class="Tbl (严格)"("Disabled"=w4816) -> ()  [unwired: 2 in, 2 out]
                n3185 = property on="加热控制参数" class="Clust (严格)"("Disabled"=2) -> ()  [unwired: 2 in, 2 out]
                n3186 = global read "功能码全局.vi" "15"() -> (w4823:bool[])
                n3187 = Index Array(array=w4823, index #1=0 ("索引"), index #2=4 ("索引")) -> (element #1=w4821:bool, element #2=w4820:bool)
                n3188 = Not(x=w4814) -> (.not. x?=w4827:bool)
              }
              frame "通道电压节数" {
                w4849 = FALSE ("1 6")
                n3189 = property on="从板号" class="DigNum (严格)"("NumText.BGColor"=u32 16777215) -> ()  [unwired: 2 in, 2 out]
                n3190 = control-ref of="项目信息 2"() -> (w4860:refnum<vi>)
                n3191 = stacked-sequence {
                  tunnel: w4860 -> [w4867 w4869 w4878]
                  frame #0 {
                    n3192 = Bundle(22, 0) -> (w4866:cluster{i32, i32})  [unwired: 1 out]
                    n3193 = property class="Tbl (严格)"(reference=w4867, "Index Values"=w4866) -> ()  [unwired: 1 in, 2 out]
                  }
                  frame #1 {
                    n3194 = for {
                      N: 40 -> [_]
                      tunnel: w4869 -> [w4876]
                      i -> [w4871]
                      n3195 = Compound Arithmetic op=ADD(0 ("值"), w4871) -> (w4873:i32)
                      n3196 = Bundle(w4873, 0) -> (w4875:cluster{i32, i32})  [unwired: 1 out]
                      n3197 = property class="Tbl (严格)"(reference=w4876, "Active Cell"=w4875, "Cell BG Color"=u32 16448250) -> ()  [unwired: 1 in, 2 out]
                    }
                  }
                  frame #2 {
                    n3198 = for {
                      N: 5 -> [_]
                      tunnel: w4878 -> [w4885]
                      i -> [w4881]
                      n3199 = Add(x=22, y=w4881) -> (x+y=w4880:i32)
                      n3200 = Bundle(w4880, 0) -> (w4884:cluster{i32, i32})  [unwired: 1 out]
                      n3201 = property class="Tbl (严格)"(reference=w4885, "Active Cell"=w4884, "Cell BG Color"=u32 6618880) -> ()  [unwired: 1 in, 2 out]
                    }
                  }
                }
                n3202 = Select(t=0, s=w4852, f=1) -> (s? t:f=w4851:i32)
                n3203 = property on="项目信息 2" class="Tbl (严格)"("Disabled"=w4851) -> ()  [unwired: 2 in, 2 out]
                n3204 = property on="加热控制参数" class="Clust (严格)"("Disabled"=2) -> ()  [unwired: 2 in, 2 out]
                n3205 = global read "功能码全局.vi" "15"() -> (w4858:bool[])
                n3206 = Index Array(array=w4858, index #1=1 ("索引"), index #2=5 ("索引")) -> (element #1=w4856:bool, element #2=w4855:bool)
                n3207 = Not(x=w4849) -> (.not. x?=w4862:bool)
              }
              frame "保险位置" {
                w4886 = FALSE ("1 6")
                n3208 = control-ref of="项目信息 2"() -> (w4897:refnum<vi>)
                n3209 = stacked-sequence {
                  tunnel: w4897 -> [w4904 w4906 w4915]
                  frame #0 {
                    n3210 = Bundle(0, 0) -> (w4903:cluster{i32, i32})  [unwired: 1 out]
                    n3211 = property class="Tbl (严格)"(reference=w4904, "Index Values"=w4903) -> ()  [unwired: 1 in, 2 out]
                  }
                  frame #1 {
                    n3212 = for {
                      N: 40 -> [_]
                      tunnel: w4906 -> [w4913]
                      i -> [w4909]
                      n3213 = Add(x=2, y=w4909) -> (x+y=w4908:i32)
                      n3214 = Bundle(w4908, 0) -> (w4912:cluster{i32, i32})  [unwired: 1 out]
                      n3215 = property class="Tbl (严格)"(reference=w4913, "Active Cell"=w4912, "Cell BG Color"=u32 16448250) -> ()  [unwired: 1 in, 2 out]
                    }
                  }
                  frame #2 {
                    n3216 = for {
                      N: 20 -> [_]
                      tunnel: w4915 -> [w4922]
                      i -> [w4918]
                      n3217 = Add(x=2, y=w4918) -> (x+y=w4917:i32)
                      n3218 = Bundle(w4917, 0) -> (w4921:cluster{i32, i32})  [unwired: 1 out]
                      n3219 = property class="Tbl (严格)"(reference=w4922, "Active Cell"=w4921, "Cell BG Color"=u32 6618880) -> ()  [unwired: 1 in, 2 out]
                    }
                  }
                }
                n3220 = property on="从板号" class="DigNum (严格)"("NumText.BGColor"=u32 16777215) -> ()  [unwired: 2 in, 2 out]
                n3221 = Select(t=0, s=w4889, f=1) -> (s? t:f=w4888:i32)
                n3222 = property on="项目信息 2" class="Tbl (严格)"("Disabled"=w4888) -> ()  [unwired: 2 in, 2 out]
                n3223 = property on="加热控制参数" class="Clust (严格)"("Disabled"=2) -> ()  [unwired: 2 in, 2 out]
                n3224 = global read "功能码全局.vi" "15"() -> (w4895:bool[])
                n3225 = Index Array(array=w4895, index #1=2 ("索引"), index #2=6 ("索引")) -> (element #1=w4893:bool, element #2=w4892:bool)
                n3226 = Not(x=w4886) -> (.not. x?=w4899:bool)
              }
              frame "温度个数" {
                w4923 = FALSE ("1 6")
                n3227 = control-ref of="项目信息 2"() -> (w4934:refnum<vi>)
                n3228 = stacked-sequence {
                  tunnel: w4934 -> [w4941 w4942 w4952]
                  frame #0 {
                    n3229 = Bundle(0, 0) -> (w4940:cluster{i32, i32})  [unwired: 1 out]
                    n3230 = property class="Tbl (严格)"(reference=w4941, "Index Values"=w4940) -> ()  [unwired: 1 in, 2 out]
                  }
                  frame #1 {
                    n3231 = for {
                      N: 40 -> [_]
                      tunnel: w4942 -> [w4950]
                      i -> [w4945]
                      n3232 = Compound Arithmetic op=ADD(0 ("值"), w4945) -> (w4947:i32)
                      n3233 = Bundle(w4947, 0) -> (w4949:cluster{i32, i32})  [unwired: 1 out]
                      n3234 = property class="Tbl (严格)"(reference=w4950, "Active Cell"=w4949, "Cell BG Color"=u32 16448250) -> ()  [unwired: 1 in, 2 out]
                    }
                  }
                  frame #2 {
                    n3235 = for {
                      N: 1 -> [_]
                      tunnel: w4952 -> [w4959]
                      i -> [w4955]
                      n3236 = Add(x=1, y=w4955) -> (x+y=w4954:i32)
                      n3237 = Bundle(w4954, 0) -> (w4958:cluster{i32, i32})  [unwired: 1 out]
                      n3238 = property class="Tbl (严格)"(reference=w4959, "Active Cell"=w4958, "Cell BG Color"=u32 6618880) -> ()  [unwired: 1 in, 2 out]
                    }
                  }
                }
                n3239 = Select(t=0, s=w4926, f=1) -> (s? t:f=w4925:i32)
                n3240 = property on="项目信息 2" class="Tbl (严格)"("Disabled"=w4925) -> ()  [unwired: 2 in, 2 out]
                n3241 = property on="加热控制参数" class="Clust (严格)"("Disabled"=2) -> ()  [unwired: 2 in, 2 out]
                n3242 = property on="从板号" class="DigNum (严格)"("NumText.BGColor"=u32 16777215) -> ()  [unwired: 2 in, 2 out]
                n3243 = global read "功能码全局.vi" "15"() -> (w4932:bool[])
                n3244 = Index Array(array=w4932, index #1=3 ("索引"), index #2=7 ("索引")) -> (element #1=w4930:bool, element #2=w4929:bool)
                n3245 = Not(x=w4923) -> (.not. x?=w4936:bool)
              }
              frame "SOC过低", "电压不均衡", "电压过低", "电压过高", "温度不均衡", "温度过低", "温度过高", "一级故障阀值" {
                w4960 = FALSE ("1 6")
                n3246 = property on="从板号" class="DigNum (严格)"("NumText.BGColor"=u32 16777215) -> ()  [unwired: 2 in, 2 out]
                n3247 = Select(t=0, s=w4962, f=1) -> (s? t:f=w4963:i32)
                n3248 = property on="一级故障 6" class="Clust (严格)"("DisabledEnum"=w4963) -> ()  [unwired: 2 in, 2 out]
                n3249 = global read "功能码全局.vi" "18"() -> (w4969:bool[])
                n3250 = Index Array(array=w4969, index #1=2 ("索引"), index #2=5 ("索引")) -> (element #1=w4967:bool, element #2=w4966:bool)
                n3251 = Not(x=w4960) -> (.not. x?=w4971:bool)
              }
              frame "SOC过低(2)", "电压不均衡(2)", "电压过低(2)", "电压过高(2)", "二级故障阀值", "温度不均衡(2)", "温度过低(2)", "温度过高(2)" {
                w4973 = FALSE ("1 6")
                n3252 = property on="从板号" class="DigNum (严格)"("NumText.BGColor"=u32 16777215) -> ()  [unwired: 2 in, 2 out]
                n3253 = Select(t=0, s=w4976, f=1) -> (s? t:f=w4975:i32)
                n3254 = property on="一级故障 7" class="Clust (严格)"("DisabledEnum"=w4975) -> ()  [unwired: 2 in, 2 out]
                n3255 = global read "功能码全局.vi" "18"() -> (w4982:bool[])
                n3256 = Index Array(array=w4982, index #1=3 ("索引"), index #2=6 ("索引")) -> (element #1=w4980:bool, element #2=w4979:bool)
                n3257 = Not(x=w4973) -> (.not. x?=w4984:bool)
              }
              frame "SOC过低(3)", "电压不均衡(3)", "电压过低(3)", "电压过高(3)", "三级故障阀值", "温度不均衡(3)", "温度过低(3)", "温度过高(3)" {
                w4986 = FALSE ("1 6")
                n3258 = property on="从板号" class="DigNum (严格)"("NumText.BGColor"=u32 16777215) -> ()  [unwired: 2 in, 2 out]
                n3259 = Select(t=0, s=w4989, f=1) -> (s? t:f=w4988:i32)
                n3260 = property on="一级故障 8" class="Clust (严格)"("DisabledEnum"=w4988) -> ()  [unwired: 2 in, 2 out]
                n3261 = global read "功能码全局.vi" "18"() -> (w4995:bool[])
                n3262 = Index Array(array=w4995, index #1=4 ("索引"), index #2=7 ("索引")) -> (element #1=w4993:bool, element #2=w4992:bool)
                n3263 = Not(x=w4986) -> (.not. x?=w4997:bool)
              }
              frame "快换参数" {
                w4999 = FALSE ("1 6")
